vi "Master.vi"() -> ()   [LabVIEW 2015]
panel:
  in  "Stop Button":bool
  in  "Cluster":T1 {"Scan in progress" scale=0.0..100.0}
  out "Waveform Chart":dbl(graph)
  in  "acquire":bool
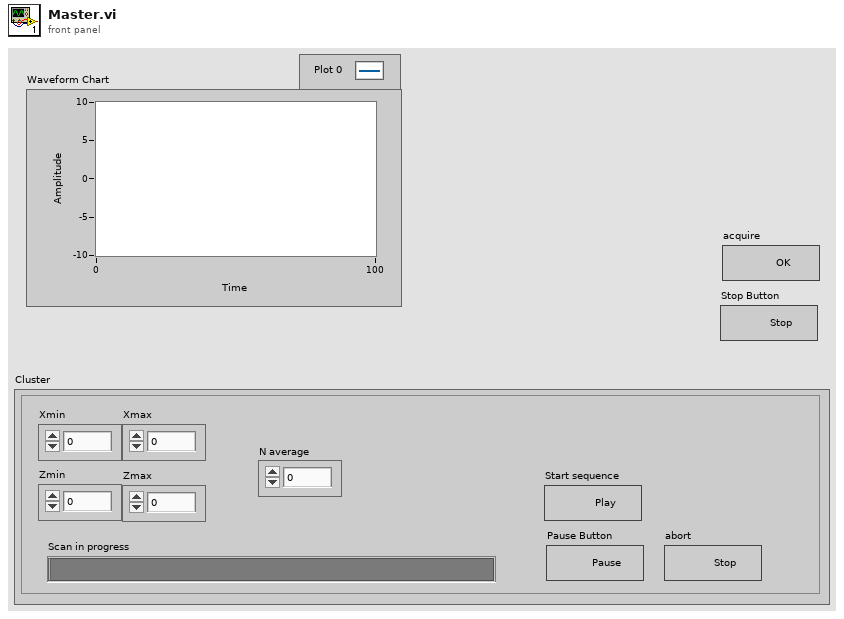
[diagram p1: front panel]
types:
  T1 = cluster{"Xmin":dbl, "Xmax":dbl, "Zmin":dbl, "Zmax":dbl, "Scan in progress":u8, "Pause Button":bool, "abort":bool, "Start sequence":bool, "N average":dbl}
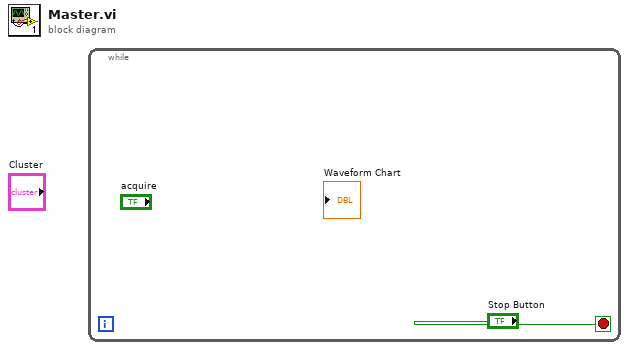
[diagram p0: block diagram]
diagram:
  n1 = while {
    stop <- "Stop Button" stop-if-true
  }
